vi "Kettle.vi"() -> ()   [LabVIEW 2020]
uses:
  <vilib>/Utility/sysdir.llb/System Directory Type.ctl
  <vilib>/Utility/file.llb/Write Delimited Spreadsheet (string).vi
panel:
  in  "Max Temp. to Stop":dbl=100.0
  in  "Outside Temperature":dbl=25.0
  out "Kettle Temp.":dbl
  in  "Kettle Condition":bool
  # "This VI is master of subVI \"Kettle Temperature.vi\". You can manage running and\nother controls from this VI. If you run this this VI, subVI will run simultaneously\n(You can observe it by placing the front panles of both VI's side by side). The value \nof \"Outside\" temperature is also the start value of kettle and when \"Kettle Condition\"\n is off this is min. value that kettle will cool down to, gradually. You can also manipulate \n\"Max Temp.\", which is considered like a safety precaution, in order to stop the VI. \n\nWhen this VI halts, it will create a CSV file on the user desktop which includes the data \noperation data of the kettle such as condition, outside temp., kettle temp and time in \neach coloumn.  If the user tries to run when CSV file is open, error will pop up. Please \nnote that if your CSV file seperators  are set to (\";\") by default, your CSV file will not be\nin order. You should either change the default settings on your computer or change \ninput \"delimiter(\\t)\" of function \"Write delimited to Spreadsheet.vi\" from (\",\") to (\";\")\n in the block diagram. And the same applies to constant input (\",\") of \"Concatenate Strings\"\nfunction."
  # "Changing default settings of seperator of CSV file on your PC(Windows 10) includes 2 \nsteps(in excel and regional settings);\n\n1)For regional settings;\n\n    -Open the Windows Start Menu and click Control Panel.\n    -Open the Regional and Language Options dialog box.\n    -Click the Regional Options tab.\n    -Click Customize/Additional settings (Windows 10)\n    -Type a comma into the 'List separator' box (\",\")\n    (You may set your decimal seperator as (\",\") and 3 digit seperator as (\".\");\n    -Click 'OK' twice to confirm the change.\n\n\n2)For excel settings;\n\n    -Click File > Options.\n    -On the Advanced tab, under Editing options, clear the Use system separators check box.\n    -Uncheck the box \"Use the system separators\", set them with the same characters\n you chose in regional then check the \n\nThen reboot your PC to see the proper operation."
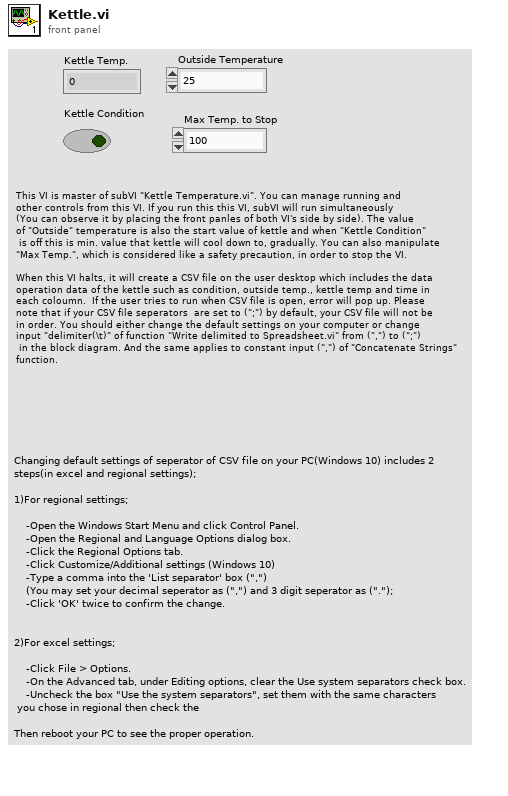
[diagram p1: front panel]
types:
  T1 = typedef "System Directory Type.ctl" = i32
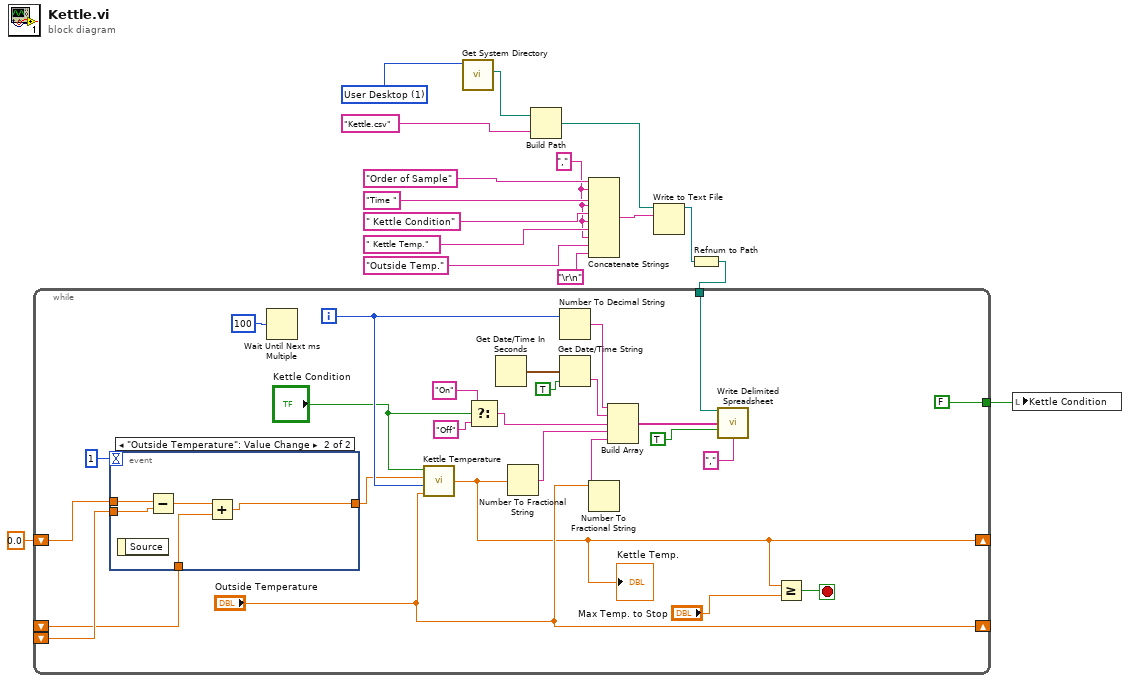
[diagram p0: block diagram]
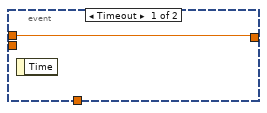
[diagram p2: hidden frame]
diagram:
  w5 = ","
  w16 = T1 1 items=["User Home"=0, "User Desktop"=1, "User Documents"=2, "User Application Data"=3, "User Preferences"=4, "User Temporary"=5, "Public Documents"=6, "Public Application Data"=7, "Public Preferences"=8, "Public Cache"=13, "System Core Libraries"=9, "System Installed Libraries"=10, "Application Files"=11, "Boot Volume Root"=12] ("system directory type")
  n1 = call <vilib>:"Get System Directory.vi"("system directory type"=w16) -> ("system directory"=w15:path)  [unwired: 10 in]
  n2 = Build Path(base path=w15, name or relative path="Kettle.csv") -> (appended path=w13:path)
  n3 = Concatenate Strings("Order of Sample", w5, "Time ", w5, " Kettle Condition" ("string"), w5, " Kettle Temp." ("string"), w5, "Outside Temp." ("string"), "\r\n") -> (w11:string)
  n4 = Write to Text File(file (use dialog)=w13, text=w11) -> (refnum out=w12:refnum<file>)  [unwired: 2 in, 2 out]
  n5 = Refnum to Path(1:w12) -> (0:w10:path)
  n6 = while {
    tunnel: w10 -> [w38]
    shift-right: [w19] -> _
    shift-left: 0.0 ("Kettle Temp.") -> [w27]
    shift-right: ["Outside Temperature"] -> _
    shift-left: _ -> [w24]
    shift-left: _ -> [w25]
    tunnel: [FALSE ("Kettle Condition")] -> w1
    i -> [w29]
    stop <- w18 stop-if-true
    n7 = event shown="[1] \"Outside Temperature\": Value Change" {
      selector: _ -> [_ _]
      dyn-events: _ -> [_ _]
      timeout: 1 -> [_ _]
      tunnel: [w43 w44] -> w26
      tunnel: w27 -> [w43 w48]
      tunnel: w25 -> [_ w47]
      tunnel: w24 -> [_ w46]
      event Timeout {
        n8 = event-data() -> ()  [unwired: 1 in, 1 out]
      }
      event "Outside Temperature": Value Change {
        n9 = event-data() -> ()  [unwired: 1 in, 1 out]
        n10 = Subtract(x=w48, y=w47) -> (x-y=w45:dbl)
        n11 = Add(x=w45, y=w46) -> (x+y=w44:dbl)
      }
    }
    n12 = Wait Until Next ms Multiple(millisecond multiple=u32 100) -> ()  [unwired: 1 out]
    n13 = call "Kettle Temperature.vi"("Outside Temp"="Outside Temperature", "Buffer(iteration)"=w29, "Buffer(Kettle Temp.)"=w26, "Kettle Condition"="Kettle Condition") -> ("Kettle Temp."=w19:dbl)
    "Kettle Temp." <- w19
    n14 = Select(t="On" ("delimiter (\\t)"), s="Kettle Condition", f="Off" ("delimiter (\\t)")) -> (s? t:f=w31:string)
    n15 = Get Date/Time In Seconds() -> (seconds since 1Jan1904=w33:timestamp)
    n16 = Number To Fractional String(number=w19) -> (F-format string=w30:string)  [unwired: 3 in]
    n17 = Number To Decimal String(number=w29) -> (decimal integer string=w36:string)  [unwired: 1 in]
    n18 = Get Date/Time String(seconds (now)=w33, want seconds? (F)=TRUE) -> (time string=w37:string)  [unwired: 1 in, 1 out]
    n19 = Number To Fractional String(number="Outside Temperature") -> (F-format string=w40:string)  [unwired: 3 in]
    n20 = Build Array(w36, w37, w31, w30, w40) -> (w39:string[])
    n21 = call-poly <vilib>:"Write Delimited Spreadsheet.vi"("file path (dialog if empty)"=w38, "1D data"=w39, "append to file? (new file:F)"=TRUE ("append to file? (F)"), "delimiter (\\t)"="," ("delimiter (\\t)")) -> ()  [unwired: 10 in, 2 out]
    n22 = Greater Or Equal?(x=w19, y="Max Temp. to Stop") -> (x >= y?=w18:bool)
  }
  n23 = local write "Kettle Condition"(w1) -> ()
